vi "Init.vi"(8 "error in (no error)":errorcluster) -> (0 "error out":errorcluster, 3 "Mock Voltage Output Out":refnum<class "Mock Voltage Output.lvclass">)   [LabVIEW 2020, in "High Level PSU With Tests.lvlib" / "Mock Voltage Output.lvclass"]
uses:
  Mock Voltage Output/Mock Voltage Output.lvclass
  Mock Voltage Output/Mock Voltage Output.lvclass/Mock Voltage Output.ctl
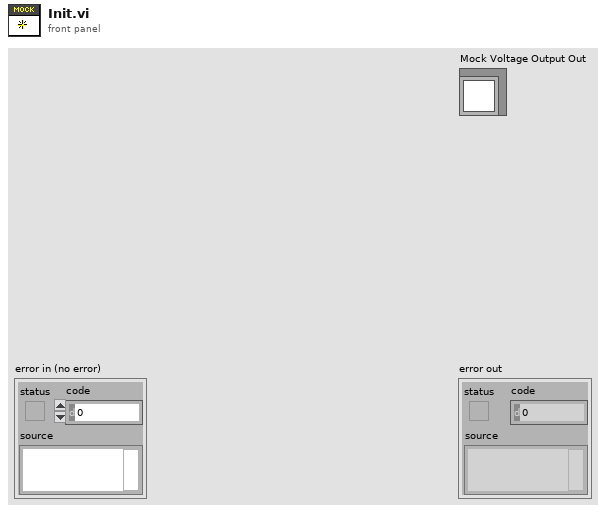
[diagram p1: front panel]
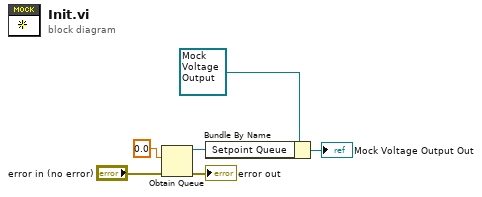
[diagram p0: block diagram]
diagram:
  n1 = Obtain Queue(element data type=0.0, error in (no error)="error in (no error)") -> (queue out=w1:refnum<queue>, error out=→"error out":errorcluster)  [unwired: 3 in, 1 out]
  n2 = Bundle By Name(cluster=refnum<class "Mock Voltage Output.lvclass"> refnum ("Mock Voltage Output In"), "Setpoint Queue"=w1) -> (→"Mock Voltage Output Out":refnum<class "Mock Voltage Output.lvclass">)
